vi "Trial Transition Logic.vi"(4 "Completed Trial Index":i32, 5 "Allow skipping":bool, 6 "Old trial index":i32, 7 "Back":bool, 8 "Subject Information":T1={" Subject"=-1, " Experiment"=0}, 9 "Num Trials":i32, 10 "Task complete":bool, 11 "Next":bool) -> (1 "New Completed Trial Index":i32, 2 "New trial index":i32)   [LabVIEW 2012]
uses:
  Experiment info.ctl
panel:
  in  "Trial Index":i32
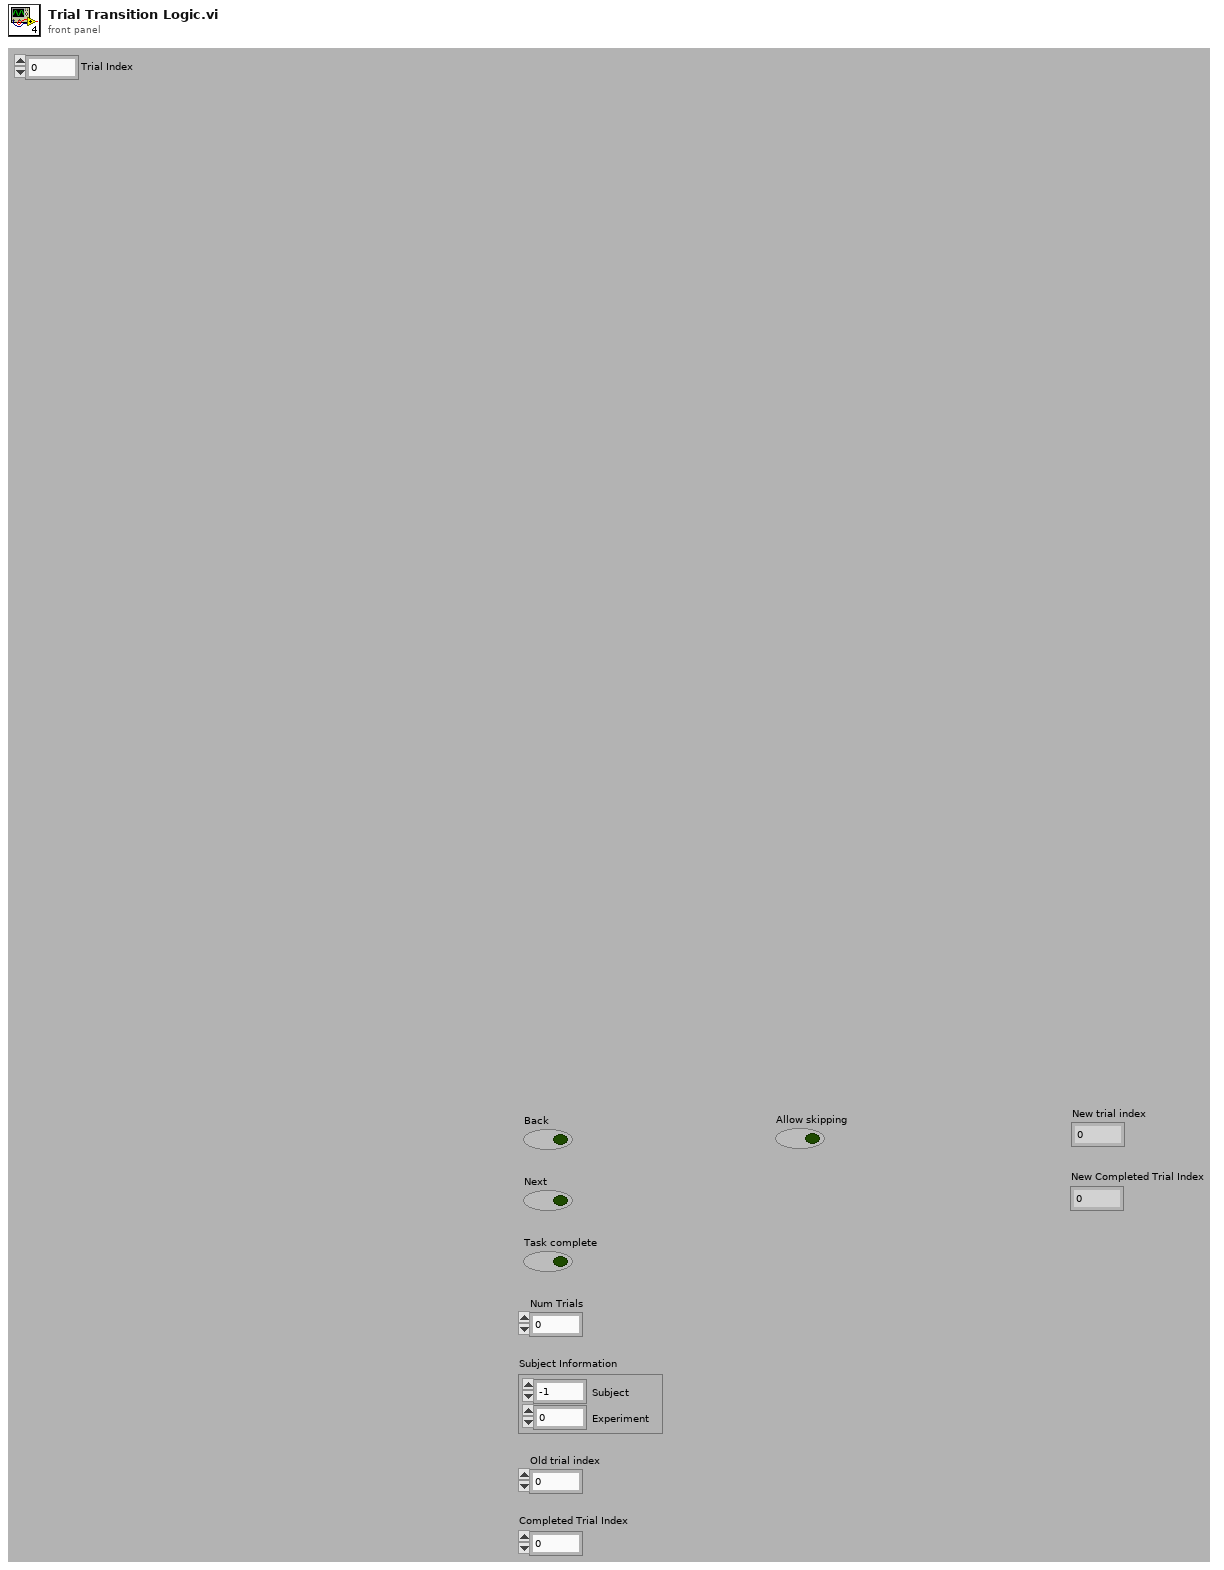
[diagram p1: front panel]
types:
  T1 = typedef "Experiment info.ctl" = cluster{" Subject":i32, " Experiment":i32}
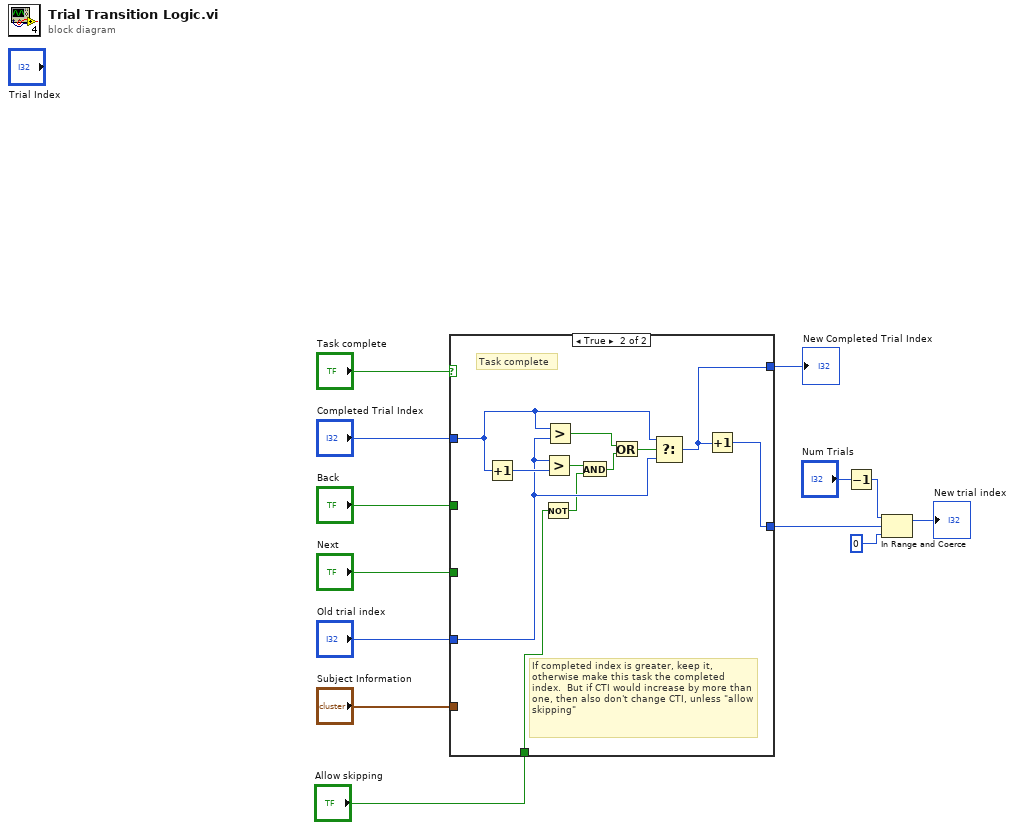
[diagram p0: block diagram]
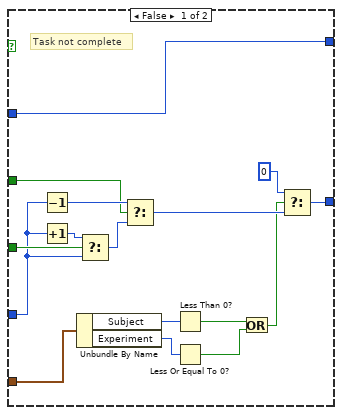
[diagram p2: hidden frame]
diagram:
  n1 = case shown="True" "Task complete" {
    tunnel: "Back" -> [w25 _]
    tunnel: "Next" -> [w24 _]
    tunnel: [w16 w40] -> w2
    tunnel: "Subject Information" -> [w23 _]
    tunnel: "Old trial index" -> [w19 w36]
    tunnel: "Completed Trial Index" -> [w17 w38]
    tunnel: [w17 w39] -> w7
    tunnel: "Allow skipping" -> [_ w30]
    frame False {
      # "Task not complete"
      n2 = Decrement(x=w19) -> (x-1=w29:i32)
      n3 = Increment(x=w19) -> (x+1=w27:i32)
      n4 = Unbundle By Name(w23) -> ("Subject"=w22:i32, "Experiment"=w21:i32)
      n5 = Select(t=w27, s=w24, f=w19) -> (s? t:f=w28:i32)
      n6 = Select(t=w29, s=w25, f=w28) -> (s? t:f=w18:i32)
      n7 = Less Than 0?(x=w22) -> (x < 0?=w26:bool)
      n8 = Less Or Equal To 0?(x=w21) -> (x <= 0?=w20:bool)
      n9 = Or(x=w26, y=w20) -> (x .or. y?=w14:bool)
      n10 = Select(t=0, s=w14, f=w18) -> (s? t:f=w16:i32)
    }
    frame True {
      # "If completed index is greater, keep it, otherwise make this task the completed index.  But if CTI would increase by more than one, then also don't change CTI, unless \"allow skipping\""
      # "Task complete"
      n11 = Increment(x=w38) -> (x+1=w37:i32)
      n12 = Not(x=w30) -> (.not. x?=w31:bool)
      n13 = Greater?(x=w36, y=w37) -> (0:w33:bool)
      n14 = Greater?(x=w38, y=w36) -> (0:w35:bool)
      n15 = And(x=w33, y=w31) -> (x .and. y?=w32:bool)
      n16 = Or(x=w35, y=w32) -> (x .or. y?=w34:bool)
      n17 = Select(t=w38, s=w34, f=w36) -> (s? t:f=w39:i32)
      n18 = Increment(x=w39) -> (x+1=w40:i32)
    }
  }
  "New Completed Trial Index" <- w7
  n19 = Decrement(x="Num Trials") -> (x-1=w6:i32)
  n20 = In Range and Coerce(upper limit=w6, x=w2, lower limit=0) -> (coerced(x)=→"New trial index":i32)  [unwired: 1 out]
